vi "From SQL Server.vi"() -> ()   [LabVIEW 2014]
uses:
  <vilib>/addons/database/NI_Database_API.lvlib
  <vilib>/addons/database/Connection.llb/DB Tools Open Connec (String).vi
  <vilib>/addons/database/Connection.llb/Conn Execute.vi
  <vilib>/addons/database/Recordset.llb/Rec Fetch Recordset Data (R).vi
  <vilib>/addons/database/Recordset.llb/Rec Destroy - Connection.vi
  <vilib>/addons/database/Connection.llb/Conn ObjectReference.ctl
panel:
  in  "停止":bool
  in  "查询":bool
  out "From SQL Server":string[][](array[string])
  out "connection reference":T1
  out "error out":errorcluster
  in  "error in (no error)":errorcluster
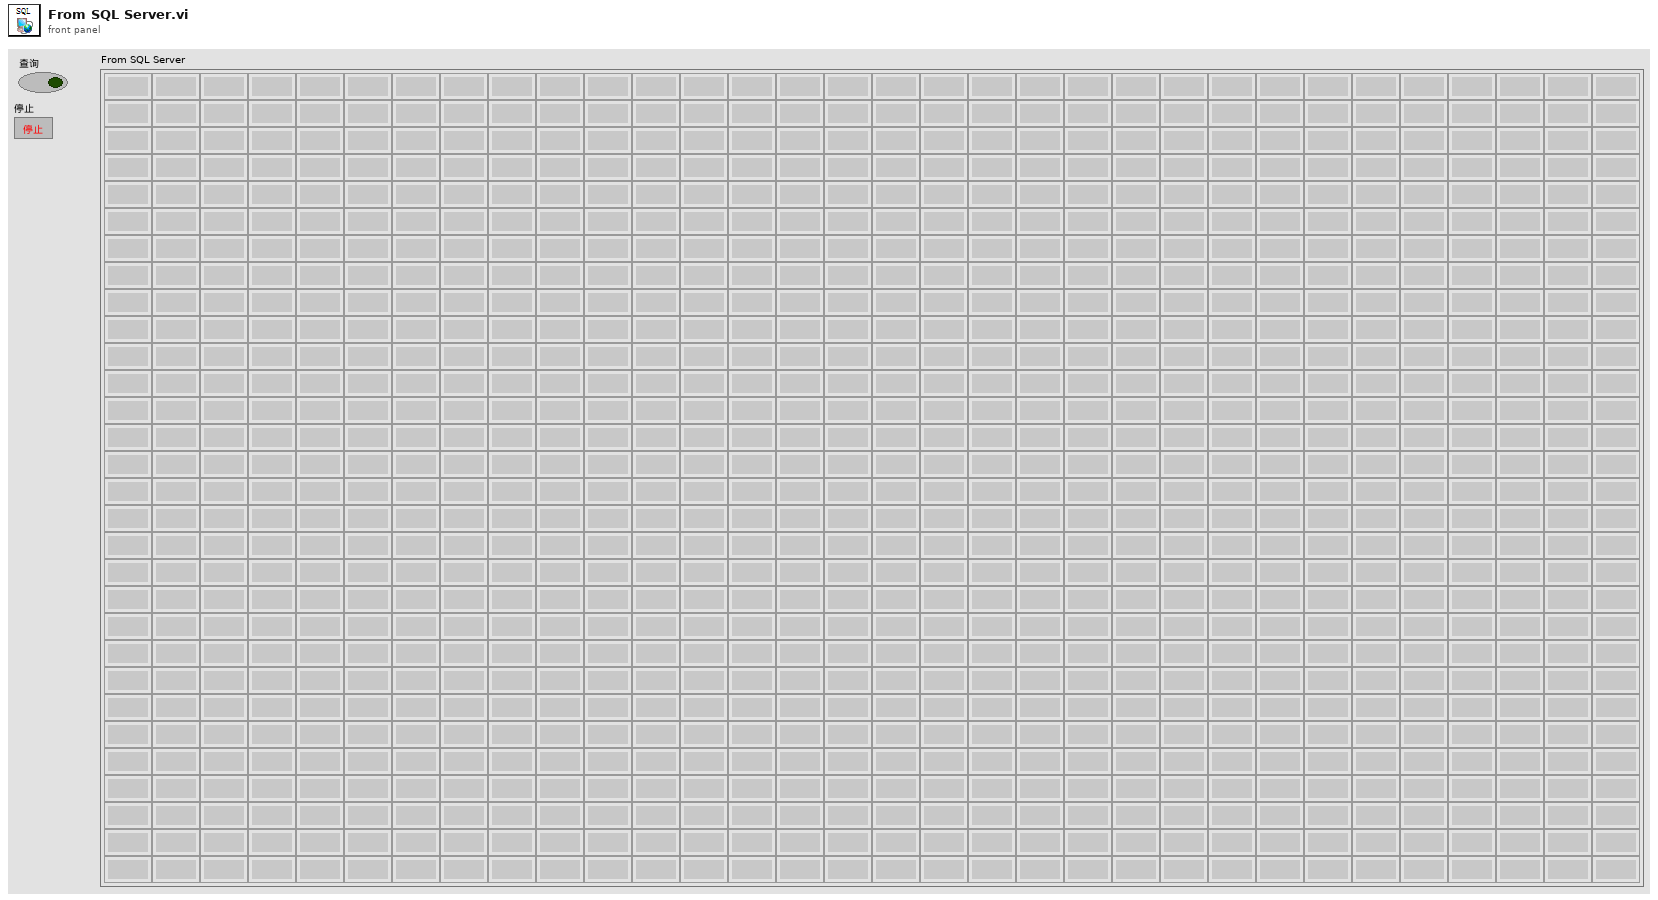
[diagram p1: front panel]
types:
  T1 = typedef "NI_Database_API.lvlib/Conn ObjectReference.ctl" = refnum<k1>
  T2 = cluster{string, string, string, string, string, string, string, string, string, string, string, string, string, string, string, string, string, string, string, string, string, string, string, string, string, string, string, string, string, string, string, string}
  T3 = typedef "NI_Database_API.lvlib/Rec ObjectReference.ctl" = refnum<k1>
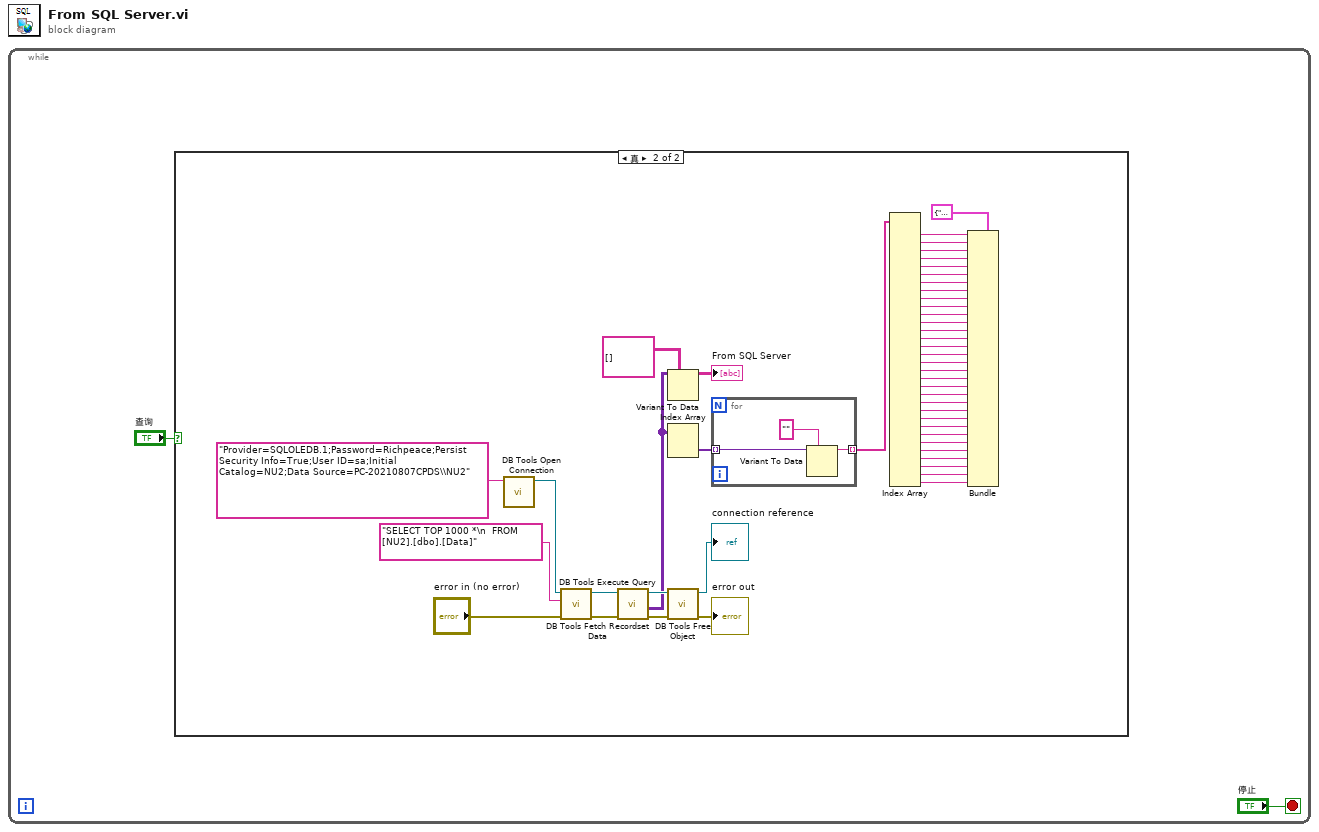
[diagram p0: block diagram]
diagram:
  n1 = while {
    stop <- "停止" stop-if-true
    n2 = case shown="真" "查询" {
      frame False {
      }
      frame True {
        n3 = call-poly <vilib>:"DB Tools Open Connection.vi"("connection information"="Provider=SQLOLEDB.1;Password=Richpeace;Persist Security Info=True;User ID=sa;Initial Catalog=NU2;Data Source=PC-20210807CPDS\\NU2" ("userID")) -> ("connection reference"=w50:T1)  [unwired: 7 in, 1 out]
        n4 = call-poly <vilib>:"DB Tools Execute Query.vi"("error in (no error)"="error in (no error)", "SQL query"="SELECT TOP 1000 *\n  FROM [NU2].[dbo].[Data]", "connection reference"=w50) -> ("error out"=w48:errorcluster, "recordset reference"=w47:T3)  [unwired: 5 in]
        n5 = call-poly <vilib>:"DB Tools Fetch Recordset Data.vi"("error in (no error)"=w48, "recordset reference"=w47) -> ("error out"=w46:errorcluster, "recordset data"=w5:variant[][], "recordset reference out"=w43:T3)  [unwired: 3 in]
        n6 = Variant To Data(type=string[][] [] ("表格控件"), Variant=w5) -> (data=→"From SQL Server":string[][])  [unwired: 1 in, 1 out]
        n7 = Index Array(array=w5) -> (element=w8:variant[])  [unwired: 2 in]
        n8 = call-poly <vilib>:"DB Tools Free Object.vi"("error in (no error)"=w46, "recordset reference"=w43) -> ("error out"=→"error out":errorcluster, "connection reference"=→"connection reference":T1)  [unwired: 8 in]
        n9 = for {
          tunnel: w8 -> [w53] mode=indexing
          tunnel: [w51] -> w7 mode=indexing
          n10 = Variant To Data(type="", Variant=w53) -> (data=w51:string)  [unwired: 1 in, 1 out]
        }
        n11 = Index Array(array=w7) -> (element #1=w40:string, element #2=w39:string, element #3=w38:string, element #4=w9:string, element #5=w10:string, element #6=w11:string, element #7=w12:string, element #8=w13:string, element #9=w14:string, element #10=w15:string, element #11=w16:string, element #12=w18:string, element #13=w17:string, element #14=w19:string, element #15=w20:string, element #16=w21:string, element #17=w22:string, element #18=w23:string, element #19=w24:string, element #20=w25:string, element #21=w26:string, element #22=w27:string, element #23=w28:string, element #24=w29:string, element #25=w30:string, element #26=w31:string, element #27=w32:string, element #28=w33:string, element #29=w34:string, element #30=w35:string, element #31=w36:string, element #32=w37:string)  [unwired: 32 in]
        n12 = Bundle(cluster=T2 {"", "", "", "", "", "", "", "", "", "", "", "", "", "", "", "", "", "", "", "", "", "", "", "", "", "", "", "", "", "", "", ""}, w40, w39, w38, w9, w10, w11, w12, w13, w14, w15, w16, w18, w17, w19, w20, w21, w22, w23, w24, w25, w26, w27, w28, w29, w30, w31, w32, w33, w34, w35, w36, w37) -> ()  [unwired: 1 out]
      }
    }
  }
